vi "GOMDBTS2048 integral Series Measure And Get Values.vi"(8 "error in (no error)":errorcluster, 10 "nrOfValues":i32, 11 "handle":i32) -> (0 "error out":errorcluster, 2 "function return":i32, 3 "integral values":dbl[](array[numeric]))   [LabVIEW 2015, in "GOMDBTS2048.lvlib"]
doc: "GOBTS2048DLL int __stdcall GOMDBTS2048_spectralGetSpectrumCalibratedPixel(int handle, double* p_spectrum);"
uses:
  GOMDBTS2048.lvlib
  runtime/GOMDBTS2048.dll
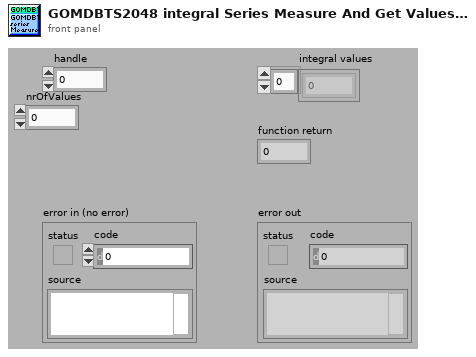
[diagram p1: front panel]
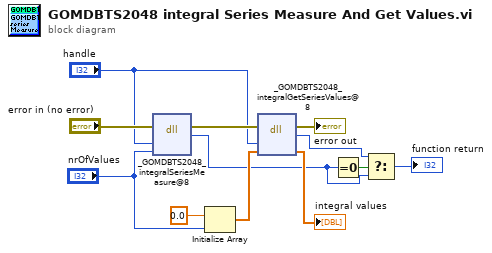
[diagram p0: block diagram]
diagram:
  n1 = dll-call lib="C:/Users/rkoch/Documents/GO_Library/runtime/GOMDBTS2048.*" fn="_GOMDBTS2048_integralSeriesMeasure@8"(error in="error in (no error)", "handle"="handle", "count"="nrOfValues") -> (error out=w7:errorcluster, "return type"=w2:i32)  [unwired: 4 in, 1 out]
  n2 = Initialize Array(0.0 ("element"), "nrOfValues") -> (w12:dbl[])
  n3 = dll-call lib="C:/Users/rkoch/Documents/GO_Library/runtime/GOMDBTS2048.*" fn="_GOMDBTS2048_integralGetSeriesValues@8"(error in=w7, "handle"="handle", "values"=w12) -> (error out=→"error out":errorcluster, "return type"=w3:i32, "values"=→"integral values":dbl[])  [unwired: 3 in, 1 out]
  n4 = Equal To 0?(x=w2) -> (x = 0?=w4:bool)
  n5 = Select(t=w3, s=w4, f=w2) -> (s? t:f=→"function return":i32)
